vi "Simulation - Tank Level Win SW demo2.vi"() -> ()   [LabVIEW 2025]
doc: "This example demonstrates a process simulation for a tank level. The process has added noise, valve deadband, lag, and deadtime. A level controller adjusts the inflow to a tank. An on/off valve serves as a drain that you can click on to operate. This s-valve represents a change in the process loading. You also can switch this VI from automatic control to manual control."
uses:
  Process.ctl
  <vilib>/addons/control/pid/pid.llb/PID Advanced (DBL).vi
  <vilib>/addons/control/pid/NI_PID_pid.lvlib
panel:
  in  "process":T1
  in  "Boolean":bool
  in  "Tab Control":enum32{"Introduction", "Operation"}(tab)=enum."Operation"
  out "Flow sensor":bool
  in  "HV-101":bool
  out "tank level":dbl(slide) scale=0.0..100.0 scale format="%#.2g"
  out "Valve":bool
  in  "LCV-101":dbl(knob) scale=0.0..100.0
  in  "Auto":bool=TRUE
  out "Process Chart":T2(graph)={"initial PV"=18.934717983735947, "SP(%)"=34.59119496855346, "output"=100.0}
  in  "Setpoint":dbl(slide)=50.0 scale=0.0..100.0
  in  "PID parameters (LIC 101)":T3={"Kc"=10.0, "Ti (min)"=0.05, "Td (min)"=0.0} {"Td (min)" format="%#.6f"; "Ti (min)" format="%#.4f"; "Kc" format="%#.4f"}
  out "flow out":dbl
  out "flow in":dbl
  in  "Stop":bool
  # "Tank Level Control"
  # "Overview: This example demonstrates a process simulation for a tank level.  The process has added noise, valve deadband, lag, and deadtime.  A level controller adjusts the inflow to a tank.  An on/off valve serves as a drain that you can click on to operate.  This s-valve represents a change in the process loading.  You also can switch this VI from automatic control to manual control.\nInstructions:\n1. Run the VI.\n2. Verify the PID controller in closed-loop to track the setpoint.\n3. Change the setpoint to another value and verify the controller tracking the new setpoint.\n4. Apply a disturbance to the system by switching the valve HV 102 (click on the valve symbol). You will see the controller recovering fro the change.\n5. Change PID gains and see if you can improve its performance without going unstable.\n6. Switch to manual mode and see if you can control the level by changing the Valve LVC 101.\n7. Click Stop to stop the VI."
  # "ISA Symbology: The diagram uses the ISA Symbology used for control"
  # "Loop 101"
  # "Level Controller at the control room"
  # "Level Transmitter on the field"
  # "Level Control Valve on the field"
  # "Hand Control Valve on the field"
  # "HV"
  # "102"
  # "LCV"
  # "101"
  # "LIC"
  # "101"
  # "LT"
  # "101"
  # "Slow Leak"
  # "Click to operate"
  # "HV"
  # "102"
  # "LCV"
  # "101"
  # "LIC"
  # "101"
  # "LT"
  # "101"
  # "Manual"
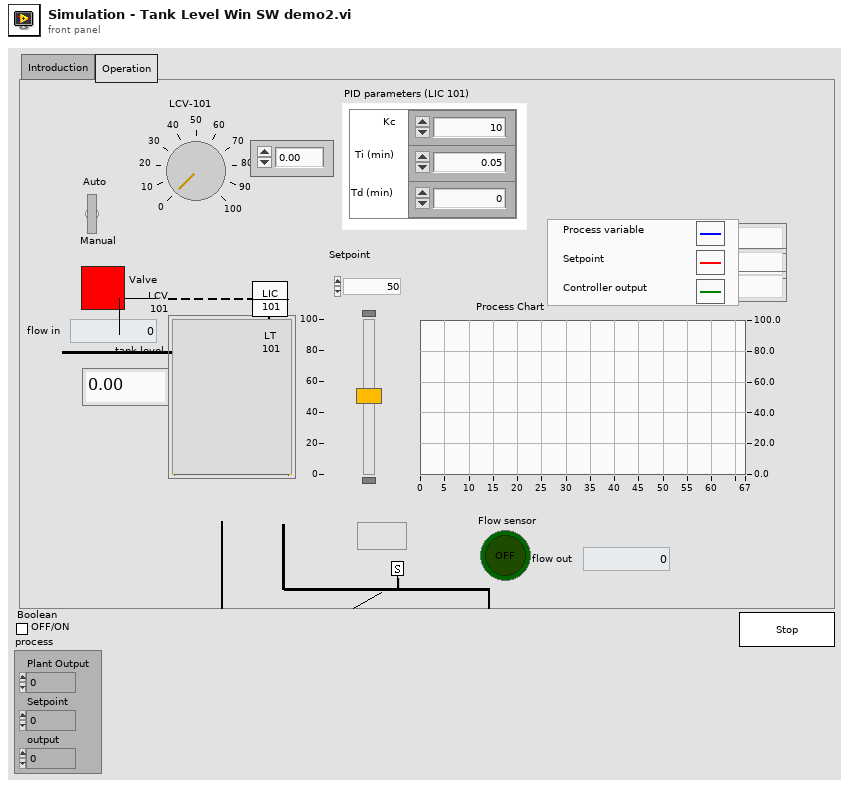
[diagram p1: front panel]
types:
  T1 = typedef "Process.ctl" = cluster{"Plant Output":dbl, "Setpoint":dbl, "output":dbl}
  T2 = cluster{"initial PV":dbl, "SP(%)":dbl, "output":dbl}
  T3 = cluster{"Kc":dbl, "Ti (min)":dbl, "Td (min)":dbl}
  T4 = cluster{"Level":dbl, "flow in":dbl, "flow out":dbl, "state_out":dbl}
  T5 = cluster{"static gain":dbl, "lag (s)":dbl, "deadtime (s)":dbl, "load":dbl, "deadband":dbl, "sensor noise":dbl, "initial PV":dbl, "plant noise":dbl}
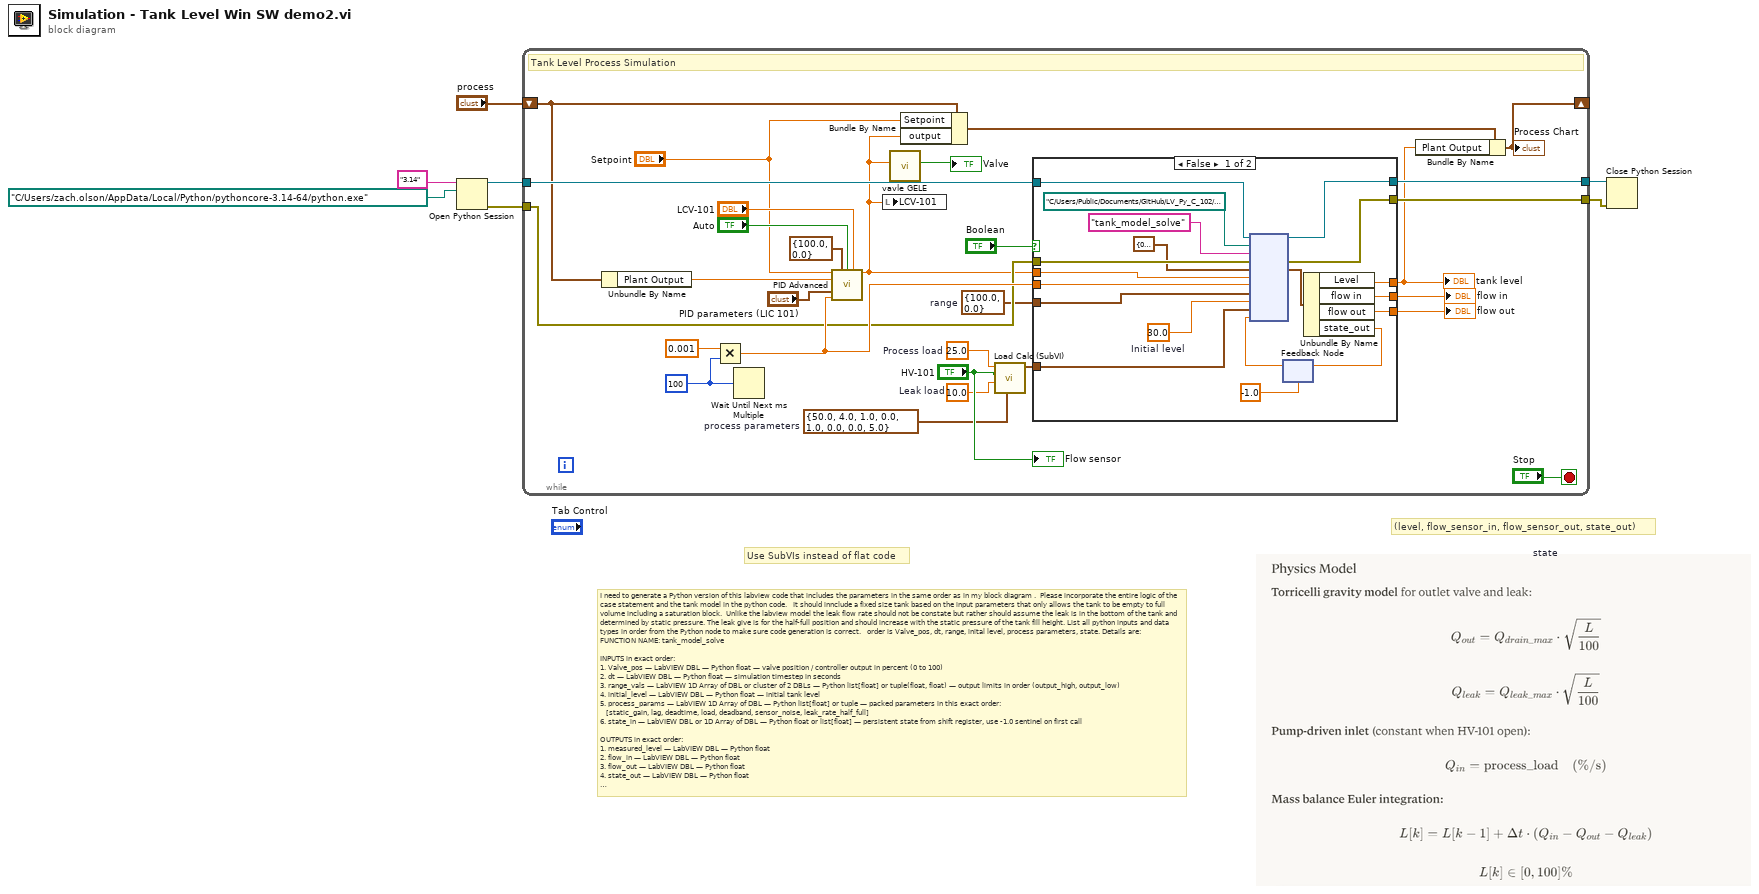
[diagram p0: block diagram]
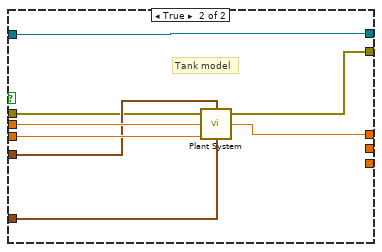
[diagram p2: hidden frame]
diagram:
  # "(level, flow_sensor_in, flow_sensor_out, state_out)"
  # "I need to generate a Python version of this labview code that includes the parameters in the same order as in my block diagram .  Please incorporate the entire logic of the case statement and the tank model in the python code.   It should innclude a fixed size tank based on the input parameters that only allows the tank to be empty to full volume including a saturation block.  Unlike the labview model the leak flow rate should not be constate but rather should assume the leak is in the bottom of the tank and determined by static pressure. The leak give is for the half-full position and should increase with the static pressure of the tank fill height. List all python inputs and data types in order from the Python node to make sure code generation is correct.   order is Valve_pos, dt, range, inital level, process parameters, state. Details are:\nFUNCTION NAME: tank_model_solve\n\nINPUTS in exact order:\n1. Valve_pos — LabVIEW DBL — Python float — valve position / controller output in percent (0 to 100)\n2. dt — LabVIEW DBL — Python float — simulation timestep in seconds\n3. range_vals — LabVIEW 1D Array of DBL or cluster of 2 DBLs — Python list[float] or tuple(float, float) — output limits in order (output_high, output_low)\n4. initial_level — LabVIEW DBL — Python float — initial tank level\n5. process_params — LabVIEW 1D Array of DBL — Python list[float] or tuple — packed parameters in this exact order:\n   [static_gain, lag, deadtime, load, deadband, sensor_noise, leak_rate_half_full]\n6. state_in — LabVIEW DBL or 1D Array of DBL — Python float or list[float] — persistent state from shift register, use -1.0 sentinel on first call\n\nOUTPUTS in exact order:\n1. measured_level — LabVIEW DBL — Python float\n2. flow_in — LabVIEW DBL — Python float\n3. flow_out — LabVIEW DBL — Python float\n4. state_out — LabVIEW DBL — Python float\n\nLabVIEW return type:\n- Cluster of 4 DBLs in the same order as the Python tuple return"
  # "Use SubVIs instead of flat code"
  n1 = Open Python Session(python version="3.14" ("Python version"), python path=path "C:/Users/zach.olson/AppData/Local/Python/pythoncore-3.14-64/python.exe" ("Python path")) -> (session out=w5:refnum<k35>, error out=w4:errorcluster)  [unwired: 1 in]
  n2 = while {
    tunnel: w5 -> [w28]
    tunnel: w4 -> [w27]
    tunnel: [w24] -> w3
    tunnel: [w23] -> w2
    shift-right: [w17] -> _
    shift-left: "process" -> [w16]
    stop <- "Stop" stop-if-true
    w10 = T5 {"static gain"=50.0, "lag (s)"=4.0, "deadtime (s)"=1.0, "load"=0.0, "deadband"=1.0, "sensor noise"=0.0, "initial PV"=0.0, "plant noise"=5.0}  # process parameters
    w25 = cluster{"output high":dbl, "output low":dbl} {"output high"=100.0, "output low"=0.0}  # range
    w13 = 25.0  # Process load
    w11 = 10.0  # Leak load
    w30 = u32 100
    # "Tank Level Process Simulation"
    n3 = Unbundle By Name(w16) -> ("Plant Output"=w15:dbl)
    n4 = Multiply(x=0.001, y=w30) -> (x*y=w29:dbl)
    n5 = Wait Until Next ms Multiple(millisecond multiple=w30) -> ()  [unwired: 1 out]
    n6 = call-poly <vilib>:"PID Advanced.vi"("setpoint"="Setpoint", "output range"=cluster{"output high":dbl, "output low":dbl} {"output high"=100.0, "output low"=0.0}, "auto? (T)"="Auto", "manual control"="LCV-101", "process variable"=w15, "PID gains"="PID parameters (LIC 101)", "dt (s)"=w29) -> ("output"=w18:dbl)  [unwired: 7 in, 1 out]
    n7 = local write "LCV-101"(w18) -> ()
    n8 = call "vavle GELE.vi"("output"=w18) -> ("T=Opening"=→"Valve":bool)  [unwired: 10 in]
    n9 = Bundle By Name(cluster=w16, "Setpoint"="Setpoint", "output"=w18) -> (w21:T1)
    n10 = call "Load Calc (SubVI).vi"("process parameters in"=w10, "Leak load"=w11, "HV-101"="HV-101", "Process load"=w13) -> ("process parameters out"=w14:T5)  [unwired: 7 in]
    n11 = case shown="False" "Boolean" {
      tunnel: w29 -> [w51 w62]
      tunnel: [w40 w61] -> w20
      tunnel: w18 -> [w52 w60]
      tunnel: w28 -> [w48 w58]
      tunnel: w27 -> [w53 w57]
      tunnel: w25 -> [w49 w59]
      tunnel: [w50 w58] -> w24
      tunnel: [w47 w57] -> w23
      tunnel: w14 -> [w45 w56]
      tunnel: [w39 _] -> w9
      tunnel: [w38 _] -> w8
      frame False {
        w46 = 30.0  # Initial level
        n12 = feedback #1 "state"(-1.0 ("output low")) -> (w43:dbl)
        n13 = node(w48, path "C:/Users/Public/Documents/GitHub/LV_Py_C_102/tank_model_solve.py" ("module path"), "tank_model_solve" ("function name"), w53, T4 {"Level"=0.0, "flow in"=0.0, "flow out"=0.0, "state_out"=0.0}, w52, w51, w49, w46, w45, w43) -> (w50:refnum<k35>, w47:errorcluster, w41:T4)  [unwired: 6 in, 2 out]
        n14 = Unbundle By Name(w41) -> ("Level"=w40:dbl, "flow in"=w39:dbl, "flow out"=w38:dbl, "state_out"=w37:dbl)
        n15 = feedback-in #1(w37) -> ()
      }
      frame True {
        # "Tank model"
        n16 = call "Plant System.vi"("output saturation range"=w59, "Plant Input"=w60, "dt (s)"=w62, "process parameters"=w56) -> ("Plant Output"=w61:dbl)  [unwired: 11 in]
      }
    }
    "tank level" <- w20
    "flow out" <- w8
    "flow in" <- w9
    n17 = Bundle By Name(cluster=w21, "Plant Output"=w20) -> (w17:T1)
    "Process Chart" <- w17
    "Flow sensor" <- "HV-101"
  }
  n18 = Close Python Session(session in=w3, error in=w2) -> ()  [unwired: 1 out]
